vi "Show Windows Task List.vi"(8 "error in (no error)":errorcluster) -> (0 "error out":errorcluster)   [LabVIEW 2023, in "Winevent.lvlib"]
doc: "This VI will show the Windows Task List.\n\nIf the Install Keyboard Filter.vi has been used to disable the Task List, this VI will not display the Task List."
uses:
  Winevent.lvlib
  WINUTIL/WINUTIL.lvlib
  user32.dll
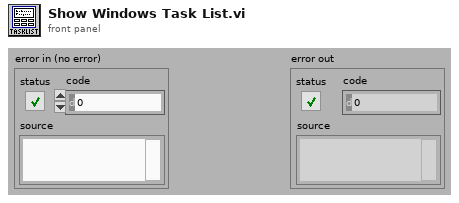
[diagram p1: front panel]
types:
  T1 = enum8{"Maximize Window", "Minimize Window", "Show Task List", "Start Screen Saver", "Quit Application"}
  T2 = typedef "WINUTIL.lvlib/Window Refnum.ctl" = refnum<k1>
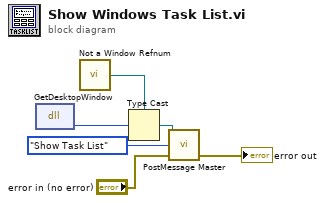
[diagram p0: block diagram]
diagram:
  n1 = dll-call lib="user32.dll" fn="GetDesktopWindow"() -> ("hWndDesktop"=w5:u32)  [unwired: 3 in, 2 out]
  n2 = call "Not a Window Refnum.vi"() -> ("Not a Window Refnum"=w4:T2)
  n3 = Type Cast(type=w4, x=w5) -> (*(type *) &x=w3:T2)
  n4 = call "PostMessage Master.vi"("window refnum"=w3, "function"=T1."Show Task List", "error in (no error)"="error in (no error)") -> ("error out"=→"error out":errorcluster)  [unwired: 1 in, 3 out]
